vi "XGT 연속읽기 Enquire.vi"(5 "명령어타입(SB)":string="SB", 6 "BCC":string, 7 "명령어(R)":string="R", 8 "데이터개수":string="02", 9 "변수이름":string="%MW000", 10 "변수길이":string="06", 11 "국번":string="0A") -> (2 "연속연결 Enquire문":string)   [LabVIEW 2014]
panel:
  in  "Header":string="\u0005"
  in  "Tail":string="\u0004"
  # "국번 10 (h0A)의 M000번지에서 부터 2개의 워드를 읽기\n\"ENQ 0A R SB 06 %MW000 02 EOT\""
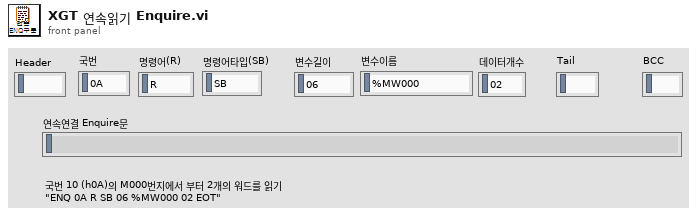
[diagram p1: front panel]
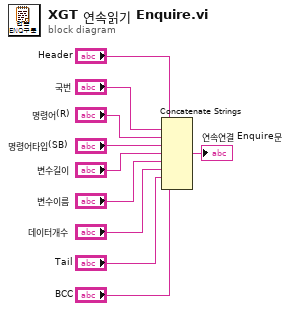
[diagram p0: block diagram]
diagram:
  n1 = Concatenate Strings("Header", "국번", "명령어(R)", "명령어타입(SB)", "변수길이", "변수이름", "데이터개수", "Tail", "BCC") -> (→"연속연결 Enquire문":string)
